vi "LVClass_CorrectionDataManager UpdateInteractionMatrix.vi"(0 "CorrectionDataManager in":refnum<class "CorrectionDataManager.lvclass">, 5 "HasoSlopes push movement":refnum<class "HasoSlopes.lvclass">, 7 "HasoSlopes pull movement":refnum<class "HasoSlopes.lvclass">, 9 "Index of actuator":i32, 11 "error in (no error)":errorcluster) -> (4 "CorrectionDataManager out":refnum<class "CorrectionDataManager.lvclass">, 15 "error out":errorcluster)   [LabVIEW 2020, in "CorrectionDataManager.lvclass"]
doc: "Update interaction matrix from two HasoSlopes resulting of one calibration\nstep for actuator index.\n\n<B>CorrDataManagerIn</B> : CorrDataManager object.\n<B>CorrDataManagerOut</B> : CorrDataManager object.\n<B>index</B> : Index of the actuator.\n<B>haso_slopes_push</B> : HasoSlopes measured for the push movement of the actuator.\n<B>haso_slopes_pull</B> : HasoSlopes measured for the pull movement of the actuator."
uses:
  CorrectionDataManager.lvclass
  HasoSlopes.lvclass
  CorrectionDataManager.lvclass/CorrectionDataManager.ctl
  LVClass_HasoSlopes Read HasoSlopes _ property.vi
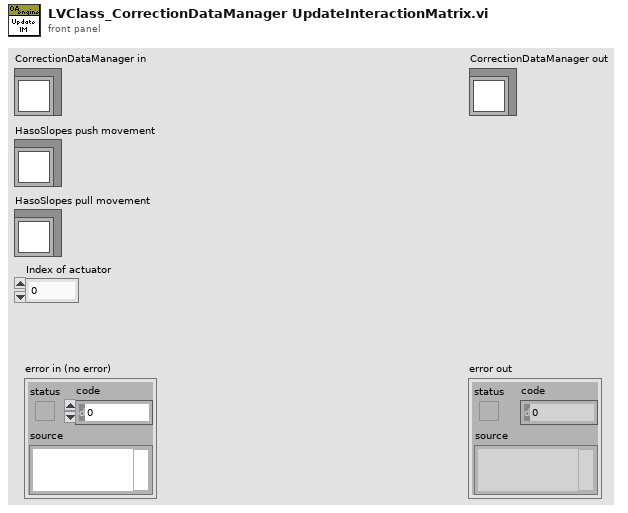
[diagram p1: front panel]
types:
  T1 = typedef "ClassID.ctl" = i64
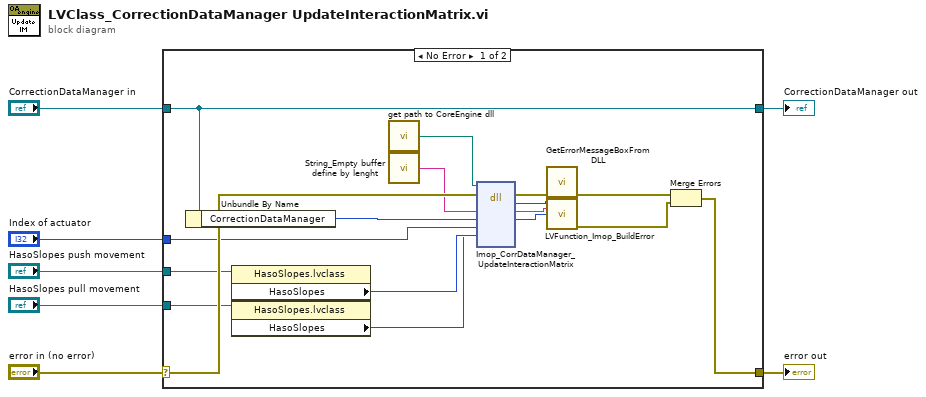
[diagram p0: block diagram]
diagram:
  n1 = case shown="No Error" "error in (no error)" {
    selector: "error in (no error)" -> [w21 w26]
    tunnel: [w22 w26] -> w6
    tunnel: [w10 w25] -> w4
    tunnel: "CorrectionDataManager in" -> [w10 w25]
    tunnel: "Index of actuator" -> [w15 _]
    tunnel: "HasoSlopes push movement" -> [w14 _]
    tunnel: "HasoSlopes pull movement" -> [w13 _]
    frame No Error {
      n2 = Unbundle By Name(w10) -> ("CorrectionDataManager"=w9:T1)
      n3 = property class="HasoSlopes.lvclass"(reference=w14) -> ("HasoSlopes"=w12:T1)  [unwired: 1 in, 2 out]
      n4 = property class="HasoSlopes.lvclass"(reference=w13) -> ("HasoSlopes"=w11:T1)  [unwired: 1 in, 2 out]
      n5 = call "get path to CoreEngine dll.vi"() -> ("path to wavekit library"=w19:path)  [unwired: 14 in, 1 out]
      n6 = call "String_Empty buffer define by lenght.vi"() -> ("Empty buffer"=w16:string)  [unwired: 1 in]
      n7 = dll-call lib="D:/FLE/0.Code/CoreEngine4_Suite/LV2011_interface/DLLs/c_interface_vc100.dll" fn="Imop_CorrDataManager_UpdateInteractionMatrix"(path in=w19, error in=w21, "Message"=w16, "Correction Data Manager"=w9, "Index of actuator"=w15, "HasoSlopes push"=w12, "Haso Slopes pull"=w11) -> (error out=w20:errorcluster, "return type"=w18:i32, "Message"=w17:string, "Correction Data Manager"=w8:i64)  [unwired: 4 in, 1 out]
      n8 = call "GetErrorMessageBoxFromDLL.vi"("error IN"=w20) -> ("error OUT"=w24:errorcluster)  [unwired: 10 in]
      n9 = call "LVFunction_Imop_BuildError.vi"("code"=w18, "String to Prepend to source (\"\")"=w17, "Adresse"=w8) -> ("error out"=w23:errorcluster)  [unwired: 12 in]
      n10 = Merge Errors(w24, w23) -> (w22:errorcluster)
    }
    frame Error {
    }
  }
  "error out" <- w6
  "CorrectionDataManager out" <- w4
